vi "Sub Initialize.vi"(8 "error in (no error)":errorcluster, 11 "RP I-V in":refnum<class "RP I-V.lvclass">) -> (0 "error out":errorcluster, 2 "Initialize Result":refnum<class "Acquired Result.lvclass">, 3 "RP I-V out":refnum<class "RP I-V.lvclass">)   [LabVIEW 2016, in "RP I-V.lvclass"]
uses:
  RP I-V.lvclass
  C:/github/LabActor/Pulse Recorders/Pulse Recorder/Pulse Recorder.lvclass
  NHMFL_Core/Libraries/Instruments/Results/Acquired Result/Acquired Result.lvclass
  NHMFL_Core/Libraries/Red Pitaya/RP Core/Rep Pitaya I-V driver/RP I-V Driver.lvclass
  C:/github/NHMFL_Core/Libraries/Instruments/Pulse Driver/Pulse Driver.lvclass
  NHMFL_Core/Libraries/Red Pitaya/RP Core/Rep Pitaya I-V driver/RP I-V Driver.lvclass/RP I-V Driver.ctl
  RP I-V.lvclass/RP I-V.ctl
  NHMFL_Core/Libraries/Red Pitaya/RP Core/Rep Pitaya I-V driver/Read Output waveform.vi
  Pulse Recorders/Pulse Recorder/Read Pulse driver.vi
  Pulse Recorders/Pulse Recorder/Write Pulse driver.vi
  Pulse Recorders/Pulse Recorder/Pulse Recorder.lvclass
  NHMFL_Core/Libraries/Instruments/Pulse Driver/Pulse Driver.lvclass
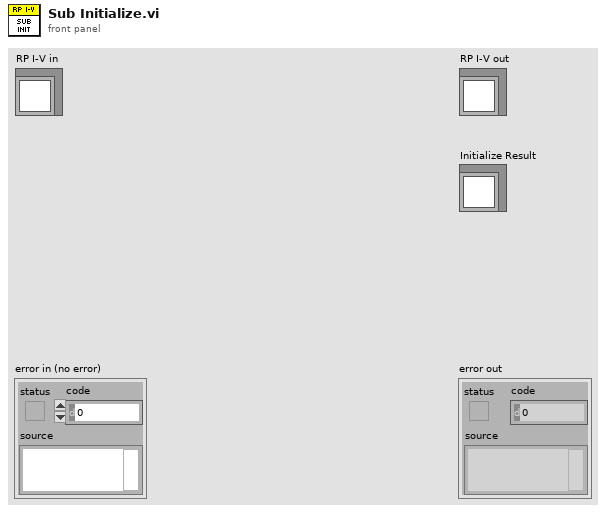
[diagram p1: front panel]
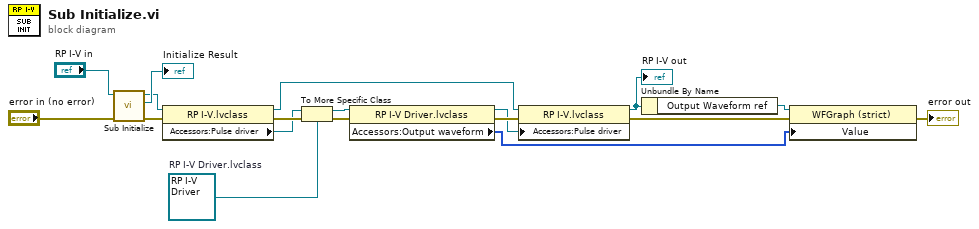
[diagram p0: block diagram]
diagram:
  w13 = refnum<class "RP I-V Driver.lvclass"> refnum  # RP I-V Driver.lvclass
  n1 = call-parent "Sub Initialize.vi"("error in (no error)"="error in (no error)", "Instrument Recorder in"="RP I-V in") -> ("error out"=w10:errorcluster, "Initialize Result"=→"Initialize Result":refnum<class "Acquired Result.lvclass">, "Instrument Recorder out"=w6:refnum<class "RP I-V.lvclass">)  [unwired: 7 in]
  n2 = property class="RP I-V.lvclass"(reference=w6, error in=w10) -> (reference out=w7:refnum<class "RP I-V.lvclass">, error out=w15:errorcluster, "Accessors:Pulse driver"=w14:refnum<class "Pulse Driver.lvclass">)
  n3 = To More Specific Class(target class=w13, reference=w14, error in=w15) -> (specific class reference=w12:refnum<class "RP I-V Driver.lvclass">, error out=w11:errorcluster)
  n4 = property class="RP I-V Driver.lvclass"(reference=w12, error in=w11) -> (reference out=w8:refnum<class "RP I-V Driver.lvclass">, error out=w9:errorcluster, "Accessors:Output waveform"=w3:i16[])
  n5 = property class="RP I-V.lvclass"(reference=w7, error in=w9, "Accessors:Pulse driver"=w8) -> (reference out=w5:refnum<class "RP I-V.lvclass">, error out=w2:errorcluster)
  "RP I-V out" <- w5
  n6 = Unbundle By Name(w5) -> ("Output Waveform ref"=w4:refnum<vi>)
  n7 = property class="WFGraph (strict)"(reference=w4, error in=w2, "Value"=w3) -> (error out=→"error out":errorcluster)  [unwired: 1 out]
